vi "Run1 Wind Turbine.vi"(11 "NXT/EV3":T1) -> (3 "EV3 out":T1)   [LabVIEW 2015]
uses:
  <vilib>/NXT/LegoClasses/BrickReference/BrickReference.lvclass
  <vilib>/NXT/Subs/LVHSConnector.ctl
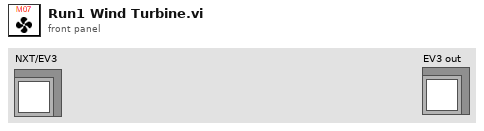
[diagram p1: front panel]
types:
  T1 = typedef "LVHSConnector.ctl" = refnum<class "BrickReference.lvclass">
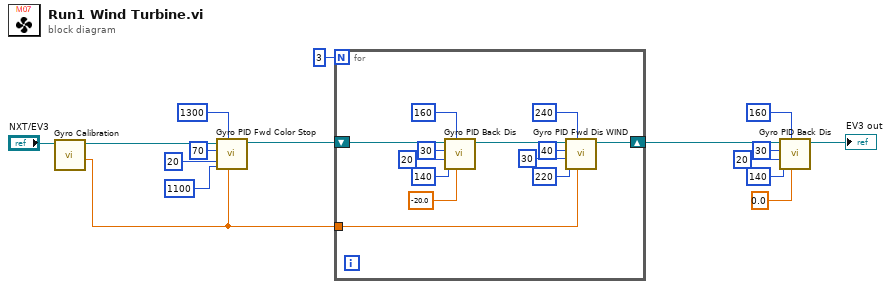
[diagram p0: block diagram]
diagram:
  n1 = call "Gyro Calibration.vi"("NXT/EV3"="NXT/EV3") -> ("Degrees"=w6:sgl, "NXT/EV3"=w16:T1)  [unwired: 6 in, 1 out]
  n2 = call "Gyro PID Fwd Color Stop.vi"("Target angle"=w6, "Threshold to Color"=1300, "Threshold to slow"=1100, "Min. speed"=20, "Max. speed"=70, "EV3 in"=w16) -> ("EV3 out"=w5:T1)  [unwired: 5 in]
  n3 = for {
    N: 3 -> [_]
    tunnel: w6 -> [w18]
    shift-right: [w19] -> w3
    shift-left: w5 -> [w17]
    n4 = call "Gyro PID Back Dis.vi"("Target angle"=sgl -20.0, "Threshold to stop"=160, "Threshold to slow"=140, "Min. speed"=20, "Max. speed"=30, "EV3 in"=w17) -> ("EV3 out"=w20:T1)  [unwired: 5 in]
    n5 = call "Gyro PID Fwd Dis WIND.vi"("Target angle"=w18, "Threshold to stop"=240, "Threshold to slow"=220, "Higher speed"=30, "Max. speed"=40, "EV3 in"=w20) -> ("EV3 out"=w19:T1)  [unwired: 5 in]
  }
  n6 = call "Gyro PID Back Dis.vi"("Target angle"=sgl 0.0, "Threshold to stop"=160, "Threshold to slow"=140, "Min. speed"=20, "Max. speed"=30, "EV3 in"=w3) -> ("EV3 out"=→"EV3 out":T1)  [unwired: 5 in]
